vi "Load_DistParts.vi"(8 "error in (no error)":errorcluster, 11 "Class in":refnum<class "IB_MSI.lvclass">) -> (0 "error out":errorcluster, 3 "Class out":refnum<class "IB_MSI.lvclass">)   [LabVIEW 2020, in "IB_MSI.lvclass"]
uses:
  <vilib>/AppBuilder/IB_Classes/MSI/IB_MSI.lvclass
  <vilib>/AppBuilder/IB_Classes/MSI/IB_MSI.lvclass/IB_MSI.ctl
  <vilib>/AppBuilder/IB_Classes/DistPart/IB_DistPart.lvclass
  <vilib>/AppBuilder/IB_Classes/Installer/Installer.lvclass
  e:/builds/penguin/labview/branches/2020/dev/dist/vi.lib/AppBuilder/IB_Classes/Installer/Installer.lvclass
  e:/builds/penguin/labview/branches/2020/dev/dist/vi.lib/AppBuilder/IB_Classes/MSI/IB_MSI.lvclass
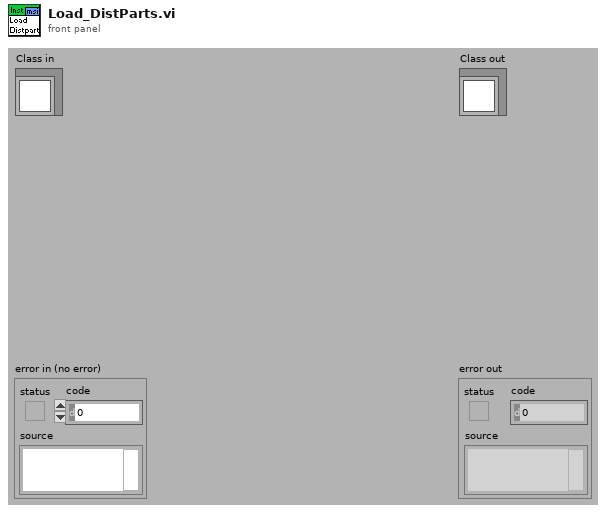
[diagram p1: front panel]
types:
  T1 = typedef "IB_Installer.ctl" = cluster{"Destination":refnum<class "IB_Destination.lvclass">[], "Source":refnum<class "IB_Source.lvclass">[], "buildObject":T2, "defaultDir":string, "platform":string, "author":string, "productName":string, "buildSpecName":string, "hide":bool, "requireLVDevSys":bool, "autoIncrement":bool, "includeError":bool, "readmeID":string, "buildLocation":path, "readmePath":path, "mediaSize":u16, "language":T3, "productVersion":T4, "preview":bool, "programmatic":bool, "progressBarEvents":T5, "userLog_Path":path, "shortcutAddresses":T7[], "EXE_Install Address":string, "EXE_Uninstall Address":string, "additional NIPaths":refnum<class "Dest_NI_NIPath.lvclass">[], "web service itemIDs":string[], "installerName":string}
  T2 = typedef "ItemRef.ctl" = u64
  T3 = typedef "CDK_sTypeDef_Languages.ctl" = u16
  T4 = typedef "CDK_sTypeDef_ProductVersion.ctl" = cluster{"Major":u8, "Minor":u8, "Update":u16}
  T5 = typedef "provcom_ProgressBar_Events.ctl" = cluster{"newJob":refnum<user-event>, "newItem":refnum<user-event>, "errorMsg":T6, "cancel":refnum<user-event>}
  T6 = typedef "mxLvBuildError.ctl" = refnum<user-event>
  T7 = typedef "CDK_sTypeDef_ShortcutAddress.ctl" = cluster{"file":string, "shortcut":string}
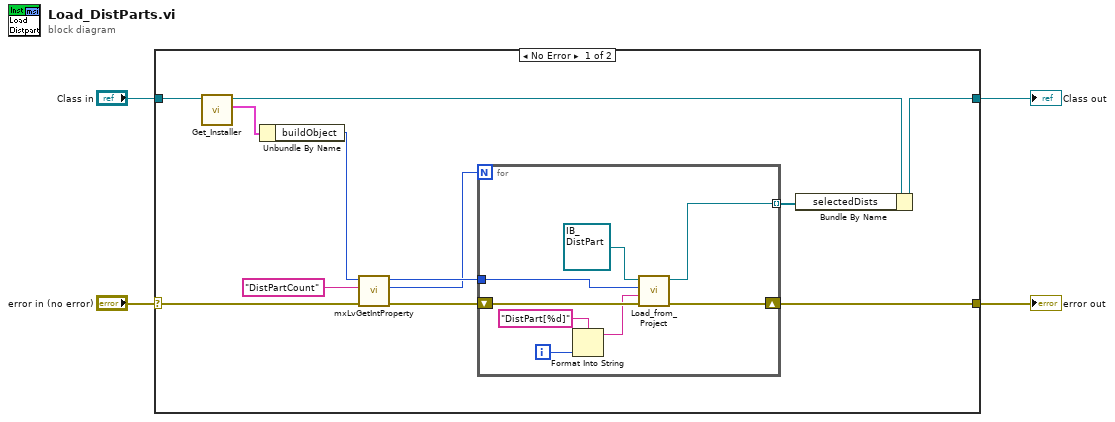
[diagram p0: block diagram]
diagram:
  n1 = case shown="No Error" "error in (no error)" {
    selector: "error in (no error)" -> [w16 w26]
    tunnel: [w15 w26] -> w3
    tunnel: [w14 w25] -> w1
    tunnel: "Class in" -> [w13 w25]
    frame No Error {
      n2 = call <vilib>:"Get_Installer.vi"("Installer in"=w13) -> ("data"=w6:T1, "Installer out"=w7:refnum<class "IB_MSI.lvclass">)  [unwired: 8 in, 1 out]
      n3 = Unbundle By Name(w6) -> ("buildObject"=w11:T2)
      n4 = call <resource>:"mxLvGetIntProperty.vi"("error in"=w16, "Tag"="DistPartCount", "Item"=w11) -> ("error out"=w8:errorcluster, "Value"=w9:i32, "Item"=w10:T2)  [unwired: 6 out]
      n5 = for {
        N: w9 -> [_]
        tunnel: w10 -> [w23]
        shift-right: [w21] -> w15
        shift-left: w8 -> [w24]
        tunnel: [w17] -> w5 mode=indexing
        i -> [w18]
        n6 = Format Into String(format string="DistPart[%d]", w18) -> (resulting string=w19:string)  [unwired: 2 in, 1 out]
        n7 = call <vilib>:"Load_from_Project.vi"("error in (no error)"=w24, "index"=w19, "buildObject"=w23, "Class in"=refnum<class "IB_DistPart.lvclass"> refnum ("IB_DistPart.lvclass")) -> ("error out"=w21:errorcluster, "Class out"=w17:refnum<class "IB_DistPart.lvclass">)  [unwired: 6 out]
      }
      n8 = Bundle By Name(cluster=w7, "selectedDists"=w5) -> (w14:refnum<class "IB_MSI.lvclass">)
    }
    frame Error {
    }
  }
  "error out" <- w3
  "Class out" <- w1
